vi "Overlay Line with Arrows Simple.vi"(6 "Color":u32(colorbox)=16711680, 7 "Group":string, 8 "error in":errorcluster, 9 "Arrows":cluster{"Start point":bool, "End point":bool}, 10 "Line Coordinates":T1, 11 "Image In":T2) -> (0 "error out":errorcluster, 3 "Image Out":T2)   [LabVIEW 2017]
uses:
  <vilib>/vision/Image Controls.llb/IMAQ Image.ctl
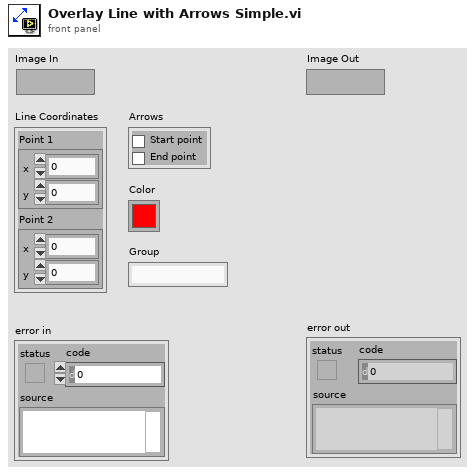
[diagram p1: front panel]
types:
  T1 = cluster{"Point 1":cluster{"x":dbl, "y":dbl}, "Point 2":cluster{"x":dbl, "y":dbl}}
  T2 = typedef "IMAQ Image.ctl" = refnum<image>
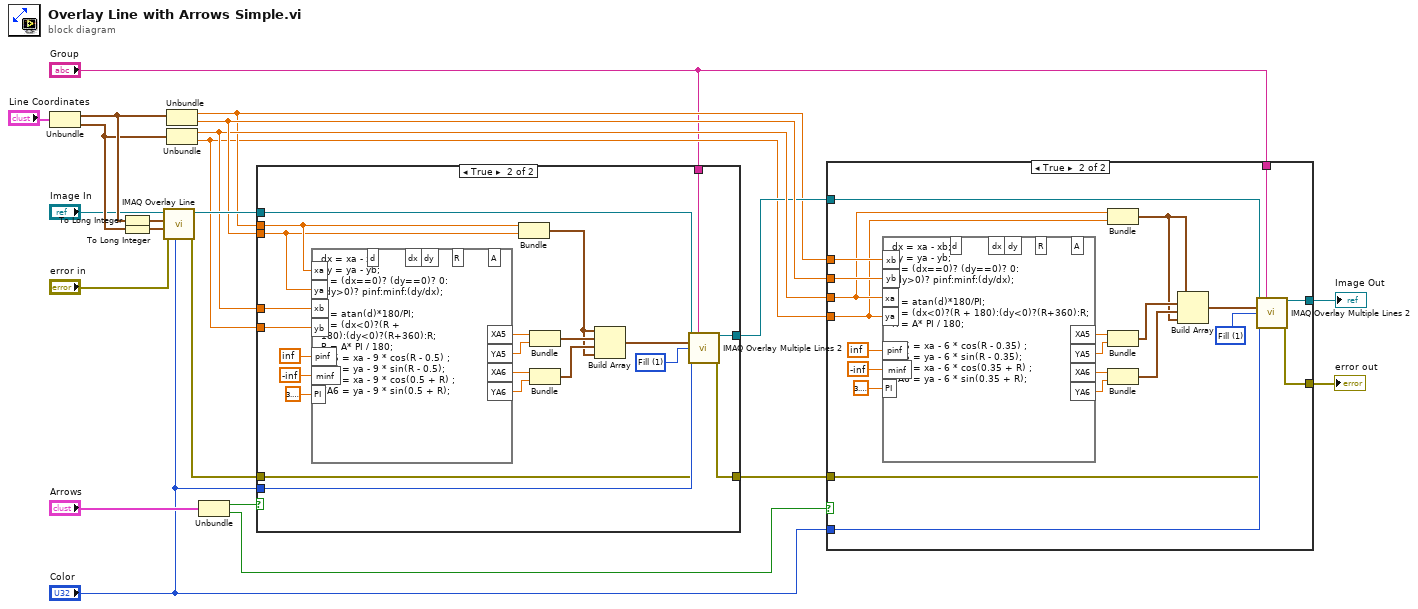
[diagram p0: block diagram]
diagram:
  n1 = Unbundle("Line Coordinates") -> ("Point 1"=w14:cluster{"x":dbl, "y":dbl}, "Point 2"=w13:cluster{"x":dbl, "y":dbl})
  n2 = To Long Integer(number=w14) -> (32bit integer=w12:cluster{"x":i32, "y":i32})
  n3 = To Long Integer(number=w13) -> (32bit integer=w11:cluster{"x":i32, "y":i32})
  n4 = call "IMAQ Overlay Line"("Color"="Color", "error in (no error)"="error in", "End Point"=w11, "Start Point"=w12, "Image"="Image In") -> ("error out"=w7:errorcluster, "Image Out"=w22:T2)  [unwired: 1 in, 4 out]
  n5 = Unbundle(w14) -> ("x"=w10:dbl, "y"=w20:dbl)
  n6 = Unbundle(w13) -> ("x"=w19:dbl, "y"=w9:dbl)
  n7 = Unbundle("Arrows") -> ("Start point"=w17:bool, "End point"=w1:bool)
  n8 = case shown="True" w17 {
    tunnel: w10 -> [_ w35]
    tunnel: w20 -> [_ w34]
    tunnel: w19 -> [_ w36]
    tunnel: w9 -> [_ w33]
    tunnel: w22 -> [w24 w32]
    tunnel: [w24 w31] -> w15
    tunnel: "Color" -> [_ w30]
    tunnel: w7 -> [w23 w28]
    tunnel: [w23 w27] -> w6
    tunnel: "Group" -> [_ w26]
    frame False {
    }
    frame True {
      w29 = u32 1 items=["Frame", "Fill"] ("Drawing Mode (Frame)")
      n9 = formula code="dx = xa - xb;\ndy = ya - yb;\nd = (dx==0)? (dy==0)? 0: \n(dy>0)? pinf:minf:(dy/dx);\n\nR = atan(d)*180/PI;\nA = (dx<0)?(R + 180):(dy<0)?(R+360):R;\nR = A* PI / 180;\nXA5 = xa - 9 * cos(R - 0.5) ;\nYA5 = ya - 9 * sin(R - 0.5);\nXA6 = xa - 9 * cos(0.5 + R) ;\nYA6 = ya - 9 * sin(0.5 + R);"("xa"=w35, "ya"=w34, "xb"=w36, "yb"=w33, "pinf"=inf, "minf"=-inf, "PI"=3.141592653589793) -> ("XA5"=w43:dbl, "YA5"=w42:dbl, "XA6"=w41:dbl, "YA6"=w40:dbl)  [unwired: 5 out]
      n10 = Bundle("x"=w35, "y"=w34) -> (w37:cluster{"x":dbl, "y":dbl})  [unwired: 1 out]
      n11 = Bundle("XA5"=w43, "YA5"=w42) -> (w39:cluster{"XA5":dbl, "YA5":dbl})  [unwired: 1 out]
      n12 = Bundle("XA6"=w41, "YA6"=w40) -> (w38:cluster{"XA6":dbl, "YA6":dbl})  [unwired: 1 out]
      n13 = Build Array(w37, w39, w38, w37) -> (w25:cluster{"x":dbl, "y":dbl}[])
      n14 = call "IMAQ Overlay Multiple Lines 2"("Image"=w32, "Group"=w26, "Line End Points"=w25, "Drawing Mode (Frame)"=w29, "Color"=w30, "error in (no error)"=w28) -> ("Image Out"=w31:T2, "error out"=w27:errorcluster)  [unwired: 8 in]
    }
  }
  n15 = case shown="True" w1 {
    tunnel: w10 -> [_ w67]
    tunnel: w20 -> [_ w66]
    tunnel: w19 -> [_ w65]
    tunnel: w9 -> [_ w64]
    tunnel: w15 -> [w48 w56]
    tunnel: [w48 w55] -> w16
    tunnel: "Color" -> [_ w54]
    tunnel: w6 -> [w47 w52]
    tunnel: [w47 w51] -> w5
    tunnel: "Group" -> [_ w50]
    frame False {
    }
    frame True {
      w53 = u32 1 items=["Frame", "Fill"] ("Drawing Mode (Frame)")
      n16 = formula code="dx = xa - xb;\ndy = ya - yb;\nd = (dx==0)? (dy==0)? 0:\n(dy>0)? pinf:minf:(dy/dx);\n\nR = atan(d)*180/PI;\nA = (dx<0)?(R + 180):(dy<0)?(R+360):R;\nR = A* PI / 180;\n\nXA5 = xa - 6 * cos(R - 0.35) ;\nYA5 = ya - 6 * sin(R - 0.35);\nXA6 = xa - 6 * cos(0.35 + R) ;\nYA6 = ya - 6 * sin(0.35 + R);"("xb"=w67, "yb"=w66, "xa"=w65, "ya"=w64, "pinf"=inf, "minf"=-inf, "PI"=3.141592653589793) -> ("XA5"=w63:dbl, "YA5"=w62:dbl, "XA6"=w61:dbl, "YA6"=w60:dbl)  [unwired: 5 out]
      n17 = Bundle("x"=w65, "y"=w64) -> (w57:cluster{"x":dbl, "y":dbl})  [unwired: 1 out]
      n18 = Bundle("XA5"=w63, "YA5"=w62) -> (w59:cluster{"XA5":dbl, "YA5":dbl})  [unwired: 1 out]
      n19 = Bundle("XA6"=w61, "YA6"=w60) -> (w58:cluster{"XA6":dbl, "YA6":dbl})  [unwired: 1 out]
      n20 = Build Array(w57, w59, w58, w57) -> (w49:cluster{"x":dbl, "y":dbl}[])
      n21 = call "IMAQ Overlay Multiple Lines 2"("Image"=w56, "Group"=w50, "Line End Points"=w49, "Drawing Mode (Frame)"=w53, "Color"=w54, "error in (no error)"=w52) -> ("Image Out"=w55:T2, "error out"=w51:errorcluster)  [unwired: 8 in]
    }
  }
  "Image Out" <- w16
  "error out" <- w5
